vi "CC Log Object.vi"(8 "error in (no error)":errorcluster, 9 "Data":variant, 10 "Source":string, 11 "Action":T1) -> (0 "error out":errorcluster, 2 "Current File":path, 3 "HK Channel out":refnum<class "HK Table.lvclass">)   [LabVIEW 2024]
uses:
  CC enum Current Values Action.ctl
  hk-channel-class/hk-channel-class/HK Table/HK Table.lvclass
  hk-channel-class/hk-channel-class/HK Table/HK Current Value Table Settings.ctl
  hk-channel-class/hk-channel-class/HK Item/HK Channel cluster Telemetry Data.ctl
  hk-channel-class/hk-channel-class/HK Item/HK Channel enum Data Type.ctl
  hk-channel-class/hk-channel-class/HK Item/HK Item.lvclass
  hk-channel-class/hk-channel-class/HK Item/HK Item.lvclass/HK Item.ctl
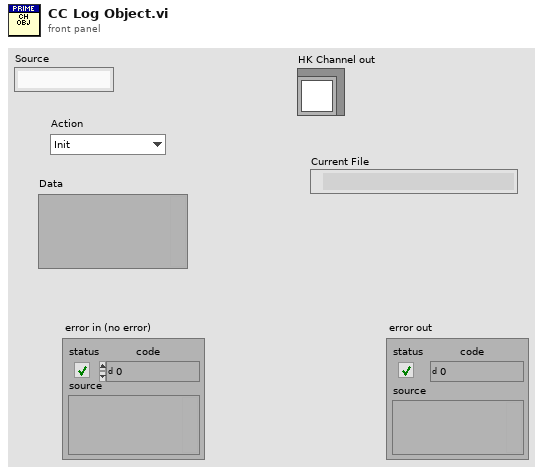
[diagram p1: front panel]
types:
  T1 = typedef "CC enum Current Values Action.ctl" = enum16{"Init", "Write Item", "Write Array", "Read Item", "Read Array", "Read All", "Add Channels", "New File", "Add Message", "Get Current Values", "Close"}
  T2 = cluster{"tdms file":refnum<k34>, "HK Channels":refnum<class "HK Table.lvclass">}
  T3 = enum16{"open", "open or create", "create or replace", "create", "open (read-only)"}
  T4 = typedef "HK Table.lvclass/HK Current Value Table Settings.ctl" = cluster{"Running Avg Elements":i32, "Max Age":dbl}
  T5 = cluster{"Name":string, "Value":dbl, "Timestamp":timestamp}
  T6 = typedef "HK Item.lvclass/HK Channel cluster Telemetry Data.ctl" = cluster{"Ch Names":string[], "Ch Values":dbl[], "Timestamp":timestamp, "Data Type":T7}
  T7 = typedef "HK Item.lvclass/HK Channel enum Data Type.ctl" = enum16{"Floating Point", "Integer", "Enum", "String", "Waveform", "File"}
  T8 = typedef "HK Table.lvclass/HK Current Value Table Element.ctl" = cluster{"Value":dbl, "Time Stamp":timestamp, "Running Avg.":dbl, "Std. Dev.":dbl, "Recent Values":dbl[], "Timestamps":timestamp[], "Alarm Status":T9}
  T9 = typedef "HK Item.lvclass/HK Alarm enum Status.ctl" = enum16{"No Alarm", "Red Low", "Red High", "Yellow Low", "Yellow High"}
  T10 = typedef "HK Item.lvclass/HK Channel Units and Setup.ctl" = cluster{"Unit Type":string, "Units":string, "Configuration":string, "Digits":i32, "Data Type":T7, "Exponential?":bool, "Source":string}
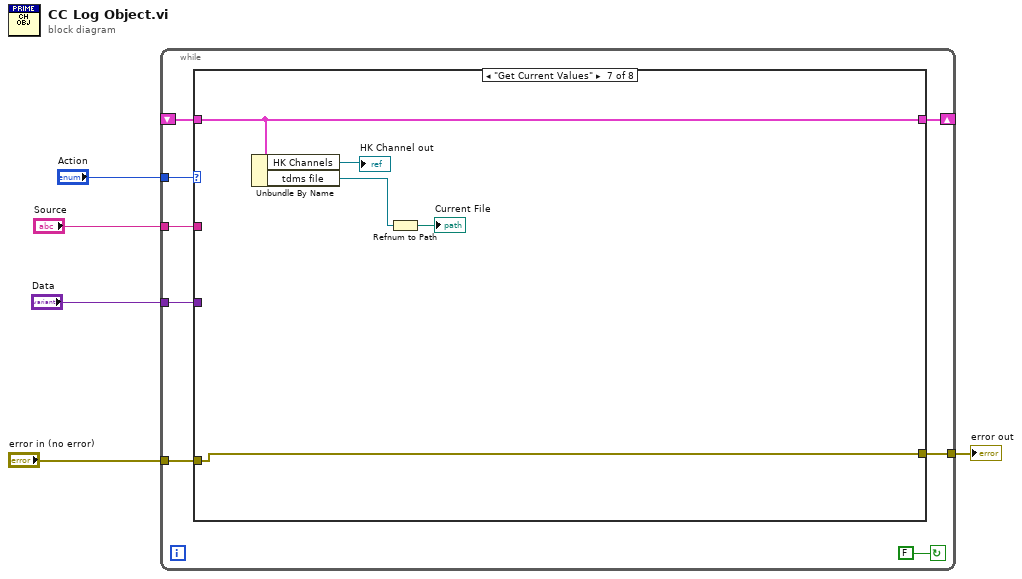
[diagram p0: block diagram]
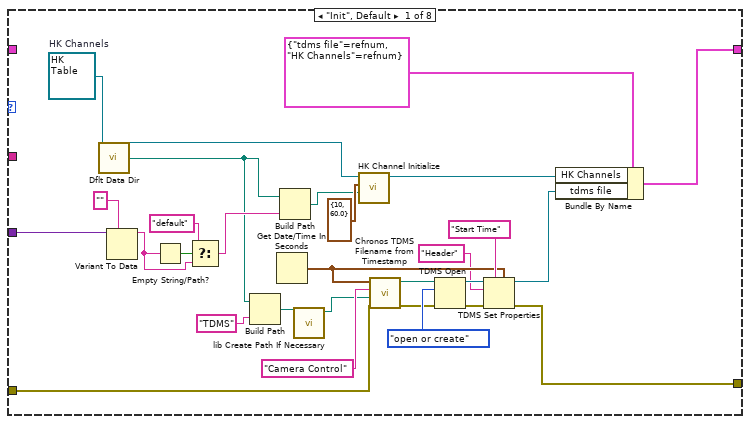
[diagram p2: hidden frame]
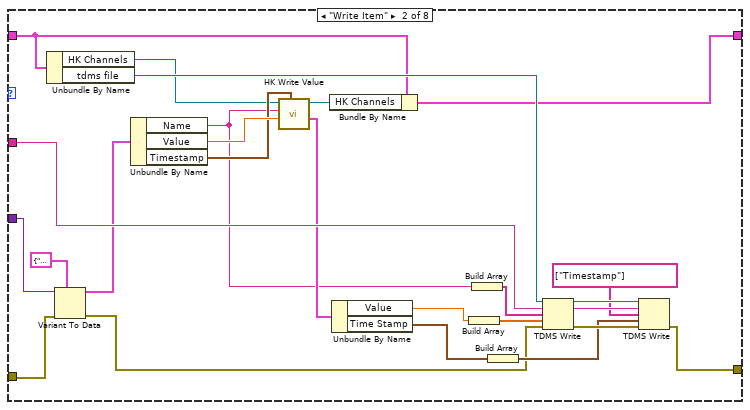
[diagram p3: hidden frame]
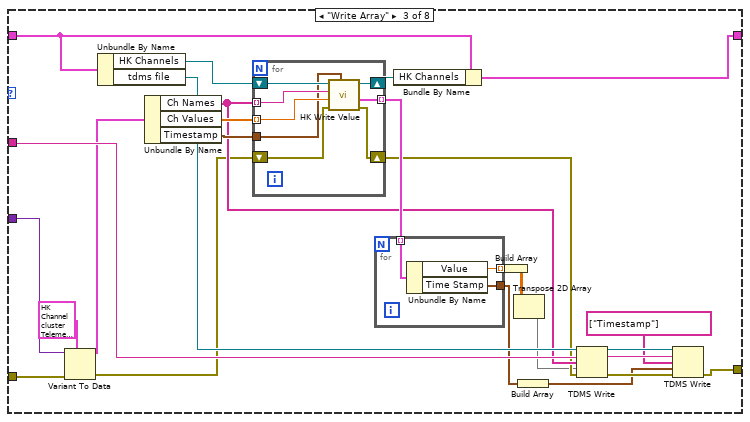
[diagram p4: hidden frame]
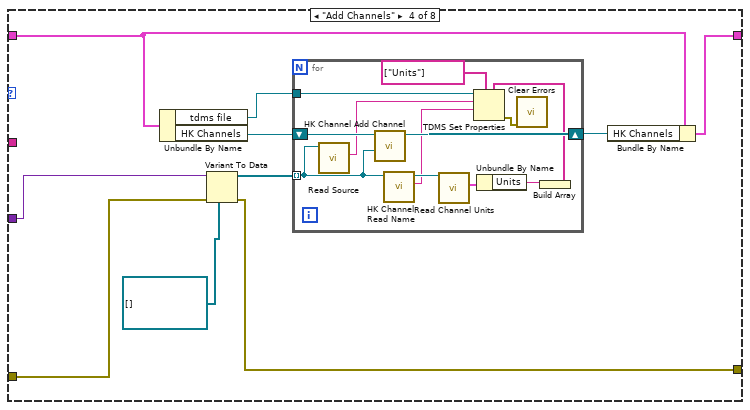
[diagram p5: hidden frame]
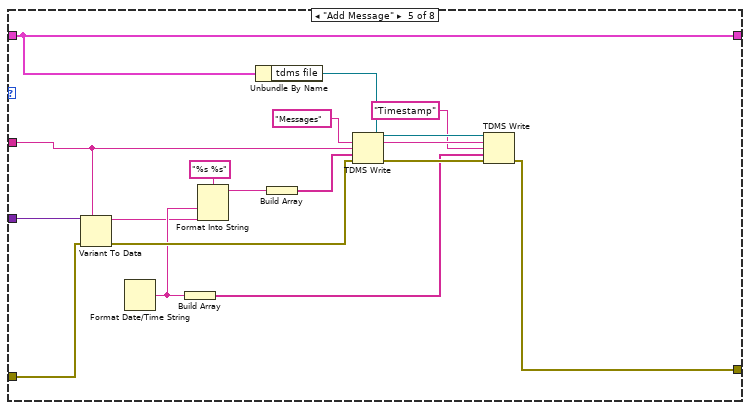
[diagram p6: hidden frame]
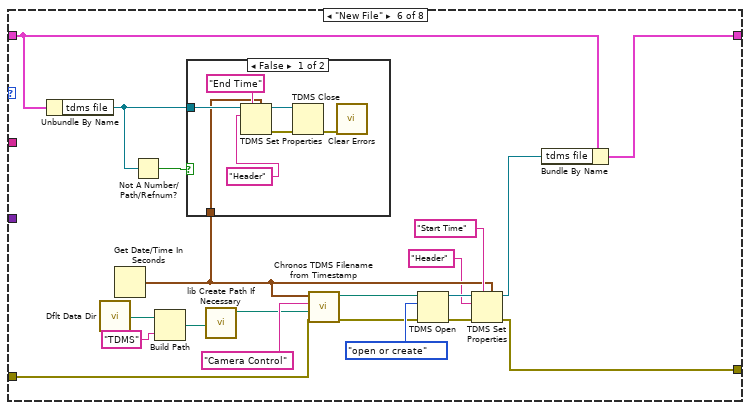
[diagram p7: hidden frame]
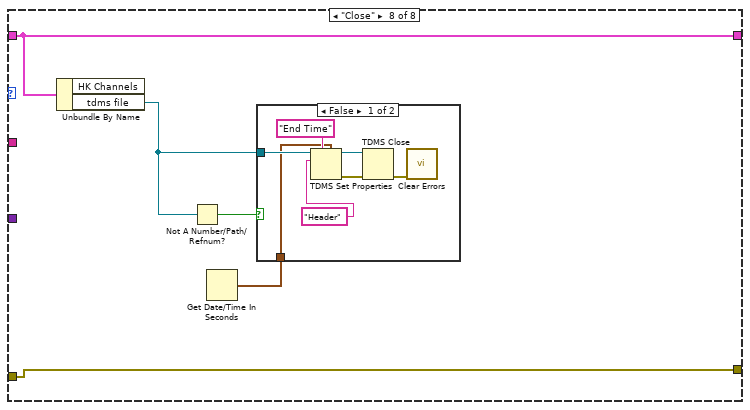
[diagram p9: hidden frame]
diagram:
  n1 = while {
    tunnel: "Action" -> [w13]
    shift-right: [w10] -> _
    shift-left: _ -> [w11]
    tunnel: "Data" -> [w9]
    tunnel: "error in (no error)" -> [w8]
    tunnel: [w7] -> w2
    tunnel: "Source" -> [w6]
    stop <- FALSE continue-if-true
    n2 = case shown="\"Get Current Values\"" w13 {
      tunnel: w11 -> [_ w47 w76 w107 w130 w158 w174 w177]
      tunnel: [w38 w48 w74 w106 w130 w157 w174 w177] -> w10
      tunnel: w9 -> [w36 w65 w92 w110 w142 _ _ _]
      tunnel: w8 -> [w31 w64 w90 w109 w132 w159 w175 w176]
      tunnel: [w27 w42 w80 w108 w131 w152 w175 w176] -> w7
      tunnel: w6 -> [_ w51 w86 _ w139 _ _ _]
      frame "Init", Default {
        w14 = refnum<class "HK Table.lvclass"> refnum  # HK Channels
        n3 = call <vilib>:"Dflt Data Dir.vi"() -> ("App:Default Data Directory"=w17:path)
        n4 = Variant To Data(type="" ("Config Name"), Variant=w36) -> (data=w22:string)  [unwired: 1 in, 1 out]
        n5 = Empty String/Path?(string/path=w22) -> (empty?=w23:bool)
        n6 = Select(t="default", s=w23, f=w22) -> (s? t:f=w20:string)
        n7 = Build Path(base path=w17, name or relative path="TDMS") -> (appended path=w18:path)
        n8 = Get Date/Time In Seconds() -> (seconds since 1Jan1904=w25:timestamp)
        n9 = Build Path(base path=w17, name or relative path=w20) -> (appended path=w39:path)
        n10 = call "lib Create Path If Necessary.vi"("path"=w18) -> ("path out"=w16:path)  [unwired: 10 in]
        n11 = call-dynamic "HK Channel Initialize.vi"("Channel Configuration File"=w39, "CVT Settings"=T4 {"Running Avg Elements"=10, "Max Age"=60.0}, "HK Channel in"=w14) -> ("HK Channel out"=w41:refnum<class "HK Table.lvclass">)  [unwired: 7 in, 1 out]
        n12 = call "Chronos TDMS Filename from Timestamp.vi"("error in (no error)"=w31, "Path to log"=w16, "suffix"="Camera Control", "time stamp"=w25) -> ("error out"=w32:errorcluster, "path"=w33:path)  [unwired: 5 in, 1 out]
        n13 = TDMS Open(8:w32, 10:T3."open or create" ("operation (0:open)"), 11:w33) -> (0:w28:errorcluster, 3:w29:refnum<k34>)  [unwired: 4 in]
        n14 = TDMS Set Properties(5:w25, 7:"Start Time", 8:w28, 10:"Header" ("group name"), 11:w29) -> (0:w27:errorcluster, 3:w26:refnum<k34>)  [unwired: 1 in, 2 out]
        n15 = Bundle By Name(cluster=T2 {"tdms file"=refnum, "HK Channels"=refnum}, "HK Channels"=w41, "tdms file"=w26) -> (w38:T2)
      }
      frame "Write Item" {
        n16 = Unbundle By Name(w47) -> ("HK Channels"=w53:refnum<class "HK Table.lvclass">, "tdms file"=w63:refnum<k34>)
        n17 = Variant To Data(error in=w64, type=T5 {"Name"="", "Value"=0.0, "Timestamp"=timestamp(0 s since 1904-01-01)}, Variant=w65) -> (data=w46:T5, error out=w43:errorcluster)
        n18 = Unbundle By Name(w46) -> ("Name"=w44:string, "Value"=w55:dbl, "Timestamp"=w54:timestamp)
        n19 = call-dynamic "HK Write Value.vi"("Timestamp"=w54, "Value"=w55, "Channel Name"=w44, "HK Channel in"=w53) -> ("value"=w45:T8, "HK Channel out"=w52:refnum<class "HK Table.lvclass">)  [unwired: 3 in, 3 out]
        n20 = Bundle By Name(cluster=w47, "HK Channels"=w52) -> (w48:T2)
        n21 = Unbundle By Name(w45) -> ("Value"=w62:dbl, "Time Stamp"=w58:timestamp)
        n22 = Build Array(w62) -> (w49:dbl[])
        n23 = Build Array(w44) -> (w50:string[])
        n24 = Build Array(w58) -> (w57:timestamp[])
        n25 = TDMS Write(0:w63, 5:w51, 7:w50, 9:w49, 11:w43) -> (4:w61:refnum<k34>, 6:w59:string, 15:w60:errorcluster)  [unwired: 1 in, 1 out]
        n26 = TDMS Write(0:w61, 5:w59, 7:string[] ["Timestamp"] ("channel name(s) in (Untitled)"), 9:w57, 11:w60) -> (15:w42:errorcluster)  [unwired: 1 in, 3 out]
      }
      frame "Write Array" {
        n27 = Variant To Data(error in=w90, type=T6 {"Ch Names"=[], "Ch Values"=[], "Timestamp"=timestamp(0 s since 1904-01-01), "Data Type"=enum."Floating Point"} ("Housekeeping Data"), Variant=w92) -> (data=w73:T6, error out=w70:errorcluster)
        n28 = Unbundle By Name(w76) -> ("HK Channels"=w77:refnum<class "HK Table.lvclass">, "tdms file"=w89:refnum<k34>)
        n29 = Unbundle By Name(w73) -> ("Ch Names"=w71:string[], "Ch Values"=w79:dbl[], "Timestamp"=w78:timestamp)
        n30 = for {
          shift-right: [w100] -> w75
          shift-left: w77 -> [w103]
          tunnel: w71 -> [w102] mode=indexing
          tunnel: w79 -> [w101] mode=indexing
          tunnel: w78 -> [w99]
          tunnel: [w98] -> w72 mode=indexing
          shift-right: [w96] -> w69
          shift-left: w70 -> [w97]
          n31 = call-dynamic "HK Write Value.vi"("Timestamp"=w99, "error in (no error)"=w97, "Value"=w101, "Channel Name"=w102, "HK Channel in"=w103) -> ("error out"=w96:errorcluster, "value"=w98:T8, "HK Channel out"=w100:refnum<class "HK Table.lvclass">)  [unwired: 2 in, 2 out]
        }
        n32 = for {
          tunnel: [w95] -> w88 mode=indexing
          tunnel: [w94] -> w83
          tunnel: w72 -> [w93] mode=indexing
          n33 = Unbundle By Name(w93) -> ("Value"=w95:dbl, "Time Stamp"=w94:timestamp)
        }
        n34 = Bundle By Name(cluster=w76, "HK Channels"=w75) -> (w74:T2)
        n35 = Build Array(w88) -> (w68:dbl[][])
        n36 = Transpose 2D Array(2D array=w68) -> (transposed array=w67:dbl[][])
        n37 = Build Array(w83) -> (w82:timestamp[])
        n38 = TDMS Write(0:w89, 5:w86, 7:w71, 9:w67, 11:w69) -> (4:w87:refnum<k34>, 6:w84:string, 15:w85:errorcluster)  [unwired: 1 in, 1 out]
        n39 = TDMS Write(0:w87, 5:w84, 7:string[] ["Timestamp"] ("channel name(s) in (Untitled)"), 9:w82, 11:w85) -> (15:w80:errorcluster)  [unwired: 1 in, 3 out]
      }
      frame "Add Channels" {
        n40 = Unbundle By Name(w107) -> ("tdms file"=w105:refnum<k34>, "HK Channels"=w113:refnum<class "HK Table.lvclass">)
        n41 = Variant To Data(error in=w109, type=refnum<class "HK Item.lvclass">[] [], Variant=w110) -> (data=w112:refnum<class "HK Item.lvclass">[], error out=w108:errorcluster)
        n42 = for {
          shift-right: [w124] -> w111
          shift-left: w113 -> [w125]
          tunnel: w112 -> [w115] mode=indexing
          tunnel: w105 -> [w123]
          n43 = call "Read Source.vi"("HK Item in"=w115) -> ("Source"=w114:string)  [unwired: 8 in, 2 out]
          n44 = call-dynamic "HK Channel Add Channel.vi"("HK Item.lvclass"=w115, "HK Channel in"=w125) -> ("HK Channel out"=w124:refnum<class "HK Table.lvclass">)  [unwired: 8 in, 1 out]
          n45 = call "HK Channel Read Name.vi"("HK Item in"=w115) -> ("Name"=w121:string, "HK Item out"=w122:refnum<class "HK Item.lvclass">)  [unwired: 8 in, 1 out]
          n46 = call "Read Channel Units.vi"("HK Item in"=w122) -> ("Channel Setup"=w120:T10)  [unwired: 8 in, 2 out]
          n47 = Unbundle By Name(w120) -> ("Units"=w118:string)
          n48 = Build Array(w118) -> (w117:string[])
          n49 = TDMS Set Properties(5:w117, 7:string[] ["Units"] ("property names"), 9:w121, 10:w114, 11:w123) -> (0:w116:errorcluster)  [unwired: 1 in, 3 out]
          n50 = call <vilib>:"Clear Errors.vi"("error in (no error)"=w116) -> ()  [unwired: 5 in, 2 out]
        }
        n51 = Bundle By Name(cluster=w107, "HK Channels"=w111) -> (w106:T2)
      }
      frame "Add Message" {
        n52 = Variant To Data(error in=w132, type=w139, Variant=w142) -> (data=w127:string, error out=w133:errorcluster)
        n53 = Format Date/Time String() -> (date/time string=w128:string)  [unwired: 3 in]
        n54 = Build Array(w128) -> (w135:string[])
        n55 = Format Into String(format string="%s %s", w128, w127) -> (resulting string=w126:string)  [unwired: 2 in, 1 out]
        n56 = Unbundle By Name(w130) -> ("tdms file"=w143:refnum<k34>)
        n57 = Build Array(w126) -> (w141:string[])
        n58 = TDMS Write(0:w143, 5:"Messages" ("group name in (Untitled)"), 7:w139, 9:w141, 11:w133) -> (4:w138:refnum<k34>, 6:w137:string, 15:w136:errorcluster)  [unwired: 1 in, 1 out]
        n59 = TDMS Write(0:w138, 5:w137, 7:"Timestamp" ("group name in (Untitled)"), 9:w135, 11:w136) -> (15:w131:errorcluster)  [unwired: 1 in, 3 out]
      }
      frame "New File" {
        n60 = Unbundle By Name(w158) -> ("tdms file"=w156:refnum<k34>)
        n61 = call <vilib>:"Dflt Data Dir.vi"() -> ("App:Default Data Directory"=w148:path)
        n62 = Get Date/Time In Seconds() -> (seconds since 1Jan1904=w149:timestamp)
        n63 = Not A Number/Path/Refnum?(number/path/refnum=w156) -> (NaN/Path/Refnum?=w155:bool)
        n64 = Build Path(base path=w148, name or relative path="TDMS") -> (appended path=w146:path)
        n65 = case shown="False" w155 {
          tunnel: w156 -> [w170 _]
          tunnel: w149 -> [w168 _]
          frame False {
            n66 = TDMS Set Properties(5:w168, 7:"End Time", 10:"Header" ("group name"), 11:w170) -> (0:w167:errorcluster, 3:w166:refnum<k34>)  [unwired: 2 in, 2 out]
            n67 = TDMS Close(8:w167, 11:w166) -> (0:w165:errorcluster)  [unwired: 1 out]
            n68 = call <vilib>:"Clear Errors.vi"("error in (no error)"=w165) -> ()  [unwired: 5 in, 2 out]
          }
          frame True {
          }
        }
        n69 = call "lib Create Path If Necessary.vi"("path"=w146) -> ("path out"=w145:path)  [unwired: 10 in]
        n70 = call "Chronos TDMS Filename from Timestamp.vi"("error in (no error)"=w159, "Path to log"=w145, "suffix"="Camera Control", "time stamp"=w149) -> ("error out"=w160:errorcluster, "path"=w161:path)  [unwired: 5 in, 1 out]
        n71 = TDMS Open(8:w160, 10:T3."open or create" ("operation (0:open)"), 11:w161) -> (0:w154:errorcluster, 3:w153:refnum<k34>)  [unwired: 4 in]
        n72 = TDMS Set Properties(5:w149, 7:"Start Time", 8:w154, 10:"Header" ("group name"), 11:w153) -> (0:w152:errorcluster, 3:w151:refnum<k34>)  [unwired: 1 in, 2 out]
        n73 = Bundle By Name(cluster=w158, "tdms file"=w151) -> (w157:T2)
      }
      frame "Get Current Values" {
        n74 = Unbundle By Name(w174) -> ("HK Channels"=→"HK Channel out":refnum<class "HK Table.lvclass">, "tdms file"=w172:refnum<k34>)
        n75 = Refnum to Path(1:w172) -> (0:→"Current File":path)
      }
      frame "Close" {
        n76 = Unbundle By Name(w177) -> ("tdms file"=w179:refnum<k34>)  [unwired: 1 out]
        n77 = Not A Number/Path/Refnum?(number/path/refnum=w179) -> (NaN/Path/Refnum?=w180:bool)
        n78 = Get Date/Time In Seconds() -> (seconds since 1Jan1904=w178:timestamp)
        n79 = case shown="False" w180 {
          tunnel: w179 -> [w187 _]
          tunnel: w178 -> [w185 _]
          frame False {
            n80 = TDMS Set Properties(5:w185, 7:"End Time", 10:"Header" ("group name"), 11:w187) -> (0:w184:errorcluster, 3:w183:refnum<k34>)  [unwired: 2 in, 2 out]
            n81 = TDMS Close(8:w184, 11:w183) -> (0:w182:errorcluster)  [unwired: 1 out]
            n82 = call <vilib>:"Clear Errors.vi"("error in (no error)"=w182) -> ()  [unwired: 5 in, 2 out]
          }
          frame True {
          }
        }
      }
    }
  }
  "error out" <- w2
